vi "ASDA-A2_Write Register Data.vi"(8 "error in":errorcluster, 10 "Write Register Data":T1 {"Min Value" format="%.0x"; "Max Value" format="%.0x"; "Address" format="%.0x"}, 11 "Buffer Data In":T2) -> (0 "error out":errorcluster, 3 "Buffer Data Out":T2)   [LabVIEW 2016]
uses:
  Data Def/ASDA-A2_Buffer Data.ctl
  Data Def/ASDA-A2_Write Register Data.ctl
  <vilib>/Modbus/master/Modbus Master.lvclass
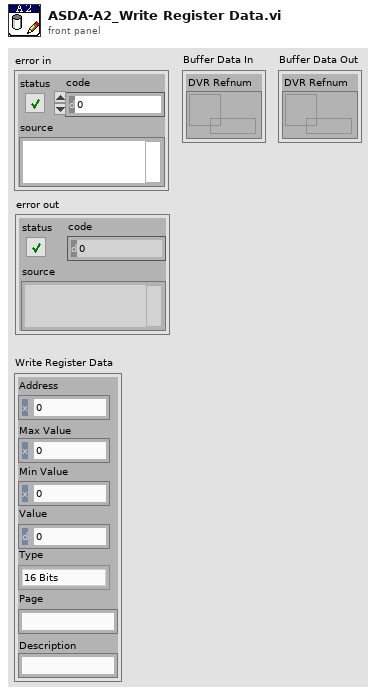
[diagram p1: front panel]
types:
  T1 = typedef "ASDA-A2_Write Register Data.ctl" = cluster{"Address":u16, "Max Value":u32, "Min Value":u32, "Value":u32, "Type":enum16{"16 Bits", "32 Bits"}, "Page":string, "Description":string}
  T2 = typedef "ASDA-A2_Buffer Data.ctl" = cluster{"DVR Refnum":refnum<data-value>}
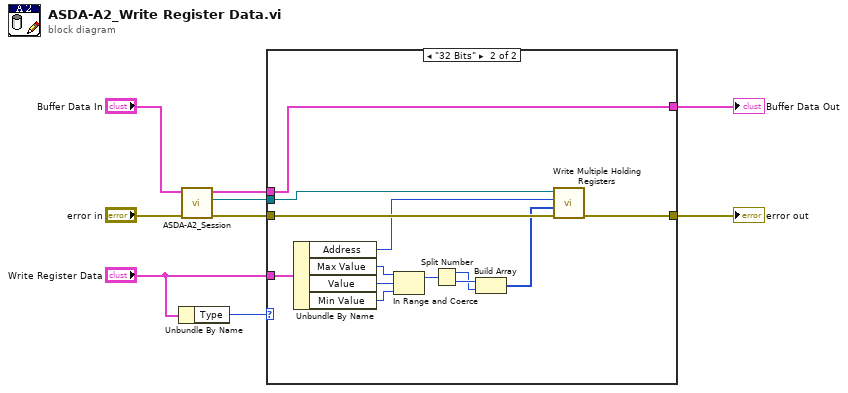
[diagram p0: block diagram]
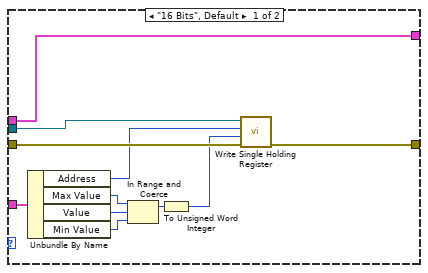
[diagram p2: hidden frame]
diagram:
  n1 = Unbundle By Name("Write Register Data") -> ("Type"=w5:enum16{"16 Bits", "32 Bits"})
  n2 = call "ASDA-A2_Session.vi"("error in"="error in", "Buffer Data In"="Buffer Data In") -> ("error out"=w7:errorcluster, "Session Out"=w6:refnum<class "Modbus Master.lvclass">, "Buffer Data Out"=w3:T2)  [unwired: 7 in]
  n3 = case shown="\"32 Bits\"" w5 {
    tunnel: w7 -> [w20 w29]
    tunnel: w6 -> [w19 w27]
    tunnel: "Write Register Data" -> [w17 w30]
    tunnel: w3 -> [w18 w28]
    tunnel: [w18 w28] -> w2
    tunnel: [w10 w25] -> w1
    frame "16 Bits", Default {
      n4 = Unbundle By Name(w17) -> ("Address"=w16:u16, "Max Value"=w13:u32, "Value"=w14:u32, "Min Value"=w15:u32)
      n5 = In Range and Coerce(upper limit=w13, x=w14, lower limit=w15) -> (coerced(x)=w12:u32)  [unwired: 1 out]
      n6 = To Unsigned Word Integer(number=w12) -> (unsigned 16bit integer=w11:u16)
      n7 = call-dynamic "Write Single Holding Register.vi"("error in (no error)"=w20, "holding register value"=w11, "address"=w16, "Modbus master in"=w19) -> ("error out"=w10:errorcluster)  [unwired: 6 in, 1 out]
    }
    frame "32 Bits" {
      n8 = Unbundle By Name(w30) -> ("Address"=w26:u16, "Max Value"=w31:u32, "Value"=w32:u32, "Min Value"=w33:u32)
      n9 = In Range and Coerce(upper limit=w31, x=w32, lower limit=w33) -> (coerced(x)=w22:u32)  [unwired: 1 out]
      n10 = Split Number(x=w22) -> (hi(x)=w23:u16, lo(x)=w24:u16)
      n11 = Build Array(w24, w23) -> (w21:u16[])
      n12 = call-dynamic "Write Multiple Holding Registers.vi"("error in (no error)"=w29, "holding register values"=w21, "starting address"=w26, "Modbus master in"=w27) -> ("error out"=w25:errorcluster)  [unwired: 6 in, 1 out]
    }
  }
  "error out" <- w1
  "Buffer Data Out" <- w2
